vi "read_waveform.vi"(8 "error in (no error)":errorcluster, 10 "Small?":bool, 11 "Dust Event ID":i32) -> (0 "error out":errorcluster, 3 "Waveform":T1)   [LabVIEW 2013]
uses:
  Controls/Waveforms.ctl
  <vilib>/addons/h5labview/H5F_mode.ctl
  Public API/Post_Signal.ctl
  Controls/Role ID.ctl
  Controls/Hardware ID.ctl
  <userlib>/_OpenG.lib/file/file.llb/File Exists - Scalar__ogtk.vi
  <vilib>/addons/h5labview/polymorph/H5A_read_var.vi
  <vilib>/addons/database/_DB Variant To Data/Database Variant To Data.xnode
  <vilib>/addons/h5labview/H5File.lvlib
  <vilib>/addons/h5labview/H5GroupObject.lvlib
  <vilib>/addons/h5labview/H5Attrib.lvlib
panel:
  out "Query Syntax":string
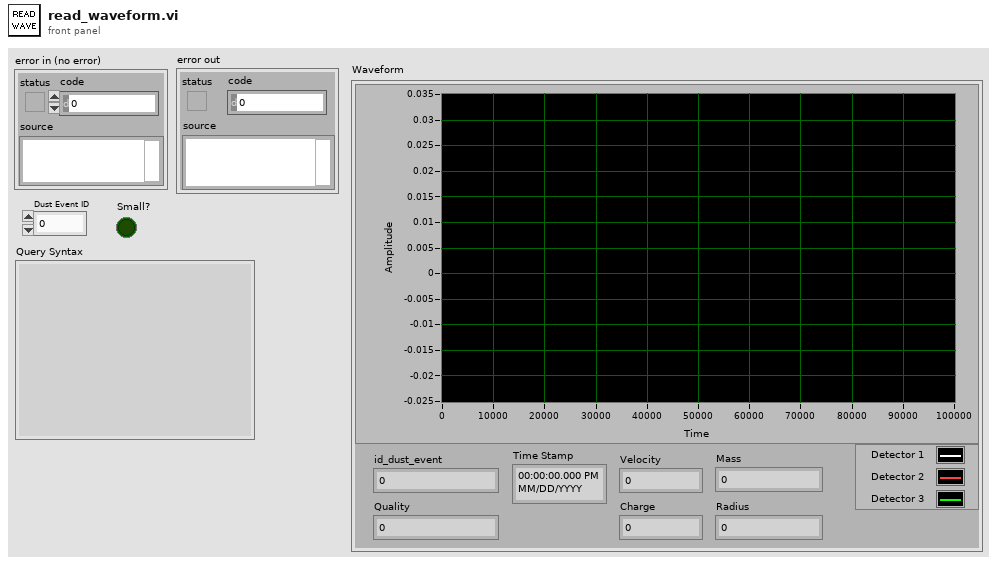
[diagram p1: front panel]
types:
  T1 = typedef "Waveforms.ctl" = cluster{"id_dust_event":u64, "Time Stamp":timestamp, "Velocity":dbl, "Mass":dbl, "Charge":dbl, "Radius":dbl, "Waveform Graph":sgl[][], "Quality":i32}
  T2 = typedef "H5File.lvlib/H5F_mode.ctl" = enum16{"read-only", "read-write", "overwrite", "create new", "open or create"}
  T3 = typedef "Role ID.ctl" = enum16{"First_Detector", "Second_Detector", "Third_Detector", "LeCroy_CH1", "LeCroy_CH2", "LeCroy_CH3", "LeCroy_CH4", "PSU"}
  T4 = typedef "Post_Signal.ctl" = cluster{"Integer Timestamp":i64, "Dust Event ID":i64, "Role ID":T3, "Data":sgl[], "Signal Length":i32, "dt":sgl, "Offset":dbl, "Hardware ID":T5}
  T5 = typedef "Hardware ID.ctl" = enum16{"Unknown", "CSA 1", "CSA 2", "CSA 3", "CSA 4", "CSA 5", "CSA 6"}
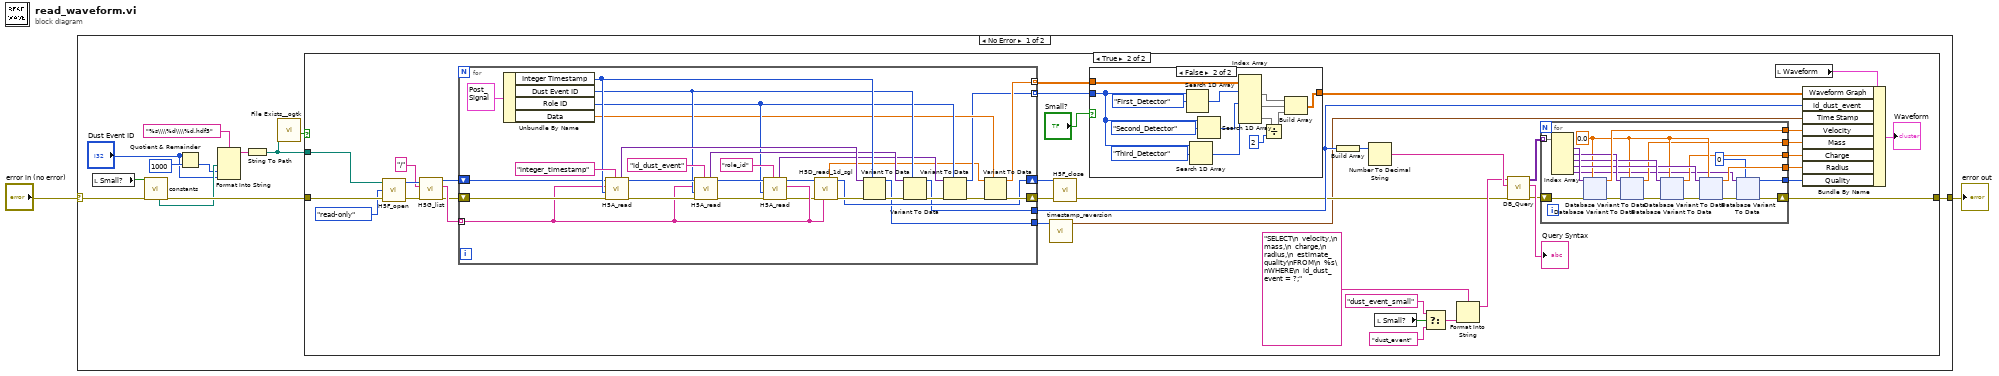
[diagram p0: block diagram]
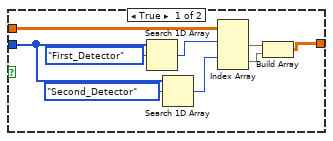
[diagram p3: hidden frame]
diagram:
  n1 = case shown="No Error" "error in (no error)" {
    selector: "error in (no error)" -> [w13 w287]
    tunnel: [w5 w287] -> w2
    frame No Error {
      n2 = local read "Small?"() -> (w6:bool)
      n3 = call "constants.vi"("error in (no error)"=w13, "Small?"=w6) -> ("error out"=w14:errorcluster, "file path for Processed Signal .hdf5 files"=w10:path)  [unwired: 4 in, 4 out]
      n4 = Quotient & Remainder(x="Dust Event ID", y=1000) -> (floor(x/y)=w9:i32)  [unwired: 1 out]
      n5 = Format Into String(format string="%s\\\\%d\\\\%d.hdf5", w10, w9, "Dust Event ID") -> (resulting string=w7:string)  [unwired: 2 in, 1 out]
      n6 = String To Path(string=w7) -> (path=w3:path)
      n7 = call-poly <userlib>:"File Exists__ogtk.vi"("file path"=w3) -> ("exists"=w4:bool)  [unwired: 6 in, 1 out]
      n8 = case shown="True" w4 {
        tunnel: w14 -> [w15 w53]
        tunnel: w3 -> [_ w52]
        tunnel: [w15 w49] -> w5
        frame False {
        }
        frame True {
          n9 = call <vilib>:"H5F_open.vi"("error in (no error)"=w53, "mode"=H5F_mode."read-only", "path"=w52) -> ("error out"=w50:errorcluster, "ref"=w48:i32)  [unwired: 1 in]
          n10 = call <vilib>:"H5G_list.vi"("error in (no error)"=w50, "group"="/", "ref"=w48) -> ("error out"=w17:errorcluster, "names"=w22:string[], "ref out"=w18:i32)  [unwired: 1 in, 1 out]
          n11 = for {
            shift-right: [w260] -> w19
            shift-left: w17 -> [w281]
            shift-right: [w259] -> w20
            shift-left: w18 -> [w282]
            tunnel: w22 -> [w265] mode=indexing
            tunnel: [w262] -> w24 mode=indexing
            tunnel: [w263] -> w25 mode=indexing
            tunnel: [w257] -> w45
            tunnel: [w258] -> w27
            n12 = Unbundle By Name(T4 {"Integer Timestamp"=0, "Dust Event ID"=0, "Role ID"=enum."First_Detector", "Data"=[], "Signal Length"=0, "dt"=0.0, "Offset"=0.0, "Hardware ID"=enum."CSA 1"} ("Post_Signal 2")) -> ("Integer Timestamp"=w284:i64, "Dust Event ID"=w276:i64, "Role ID"=w270:T3, "Data"=w267:sgl[])
            n13 = call-poly <vilib>:"H5A_read.vi"("attrib_name"="integer_timestamp", "error in (no error)"=w281, "default"=w284, "obj_name"=w265, "ref"=w282) -> ("error out"=w278:errorcluster, "ref out"=w280:i32, "value"=w283:variant)  [unwired: 2 in]
            n14 = call-poly <vilib>:"H5A_read.vi"("attrib_name"="id_dust_event", "error in (no error)"=w278, "default"=w276, "obj_name"=w265, "ref"=w280) -> ("error out"=w274:errorcluster, "ref out"=w273:i32, "value"=w277:variant)  [unwired: 2 in]
            n15 = call-poly <vilib>:"H5A_read.vi"("attrib_name"="role_id", "error in (no error)"=w274, "default"=w270, "obj_name"=w265, "ref"=w273) -> ("error out"=w264:errorcluster, "ref out"=w266:i32, "value"=w271:variant)  [unwired: 2 in]
            n16 = call "H5D_read_1d_sgl.vi"("name"=w265, "error in (no error)"=w264, "ref"=w266) -> ("error out"=w261:errorcluster, "ref out"=w259:i32, "data"=w256:sgl[])  [unwired: 4 in]
            n17 = Variant To Data(error in=w261, type=w284, Variant=w283) -> (data=w258:i64, error out=w275:errorcluster)
            n18 = Variant To Data(error in=w275, type=w276, Variant=w277) -> (data=w257:i64, error out=w269:errorcluster)
            n19 = Variant To Data(error in=w269, type=w270, Variant=w271) -> (data=w262:T3, error out=w268:errorcluster)
            n20 = Variant To Data(error in=w268, type=w267, Variant=w256) -> (data=w263:sgl[], error out=w260:errorcluster)
          }
          n21 = call "timestamp_reversion.vi"("Integer Timestamp"=w27) -> ("time stamp"=w28:timestamp)  [unwired: 8 in, 1 out]
          n22 = call <vilib>:"H5F_close.vi"("error in (no error)"=w19, "ref"=w20) -> ("error out"=w42:errorcluster)  [unwired: 3 in]
          n23 = case shown="False" "Small?" {
            tunnel: w24 -> [w238 w251]
            tunnel: w25 -> [w236 w248]
            tunnel: [w233 w245] -> w26
            frame True {
              n24 = Search 1D Array(1D array=w238, element=Role_ID."First_Detector") -> (index of element=w239:i32)  [unwired: 1 in]
              n25 = Search 1D Array(1D array=w238, element=Role_ID."Second_Detector") -> (index of element=w237:i32)  [unwired: 1 in]
              n26 = Index Array(array=w236, index (row) #1=w239, index (row) #2=w237) -> (element #1=w235:sgl[], element #2=w234:sgl[])  [unwired: 2 in]
              n27 = Build Array(w235, w234) -> (w233:sgl[][])
            }
            frame False {
              n28 = Search 1D Array(1D array=w251, element=Role_ID."First_Detector") -> (index of element=w253:i32)  [unwired: 1 in]
              n29 = Search 1D Array(1D array=w251, element=Role_ID."Third_Detector") -> (index of element=w249:i32)  [unwired: 1 in]
              n30 = Search 1D Array(1D array=w251, element=Role_ID."Second_Detector") -> (index of element=w250:i32)  [unwired: 1 in]
              n31 = Index Array(array=w248, index (row) #1=w253, index (row) #2=w250, index (row) #3=w249) -> (element #1=w247:sgl[], element #2=w246:sgl[], element #3=w244:sgl[])  [unwired: 3 in]
              n32 = Divide(x=w244, y=2 ("Numeric")) -> (x/y=w243:sgl[])
              n33 = Build Array(w247, w246, w243) -> (w245:sgl[][])
            }
          }
          n34 = Build Array(w45) -> (w46:i64[])
          n35 = Number To Decimal String(number=w46) -> (decimal integer string=w47:string[])  [unwired: 1 in]
          n36 = local read "Small?"() -> (w32:bool)
          n37 = Select(t="dust_event_small" ("resulting string"), s=w32, f="dust_event" ("resulting string")) -> (s? t:f=w31:string)
          n38 = Format Into String(format string="SELECT\n  velocity,\n  mass,\n  charge,\n  radius,\n  estimate_quality\nFROM\n  %s\nWHERE\n  id_dust_event = ?;" ("SQL query"), w31) -> (resulting string=w44:string)  [unwired: 2 in, 1 out]
          n39 = call "DB_Query.vi"("error in (no error)"=w42, "Parameters"=w47, "Parameterized Query"=w44) -> ("error out"=w40:errorcluster, "Query in Standard Format"=→"Query Syntax":string, "Results"=w41:variant[][])  [unwired: 6 in]
          n40 = for {
            tunnel: w41 -> [w71] mode=indexing
            shift-right: [w57] -> w49
            shift-left: w40 -> [w72]
            tunnel: [w68] -> w35
            tunnel: [w61] -> w36
            tunnel: [w60] -> w37
            tunnel: [w59] -> w38
            tunnel: [w54] -> w39
            w62 = 0.0 ("Velocity")
            n41 = Index Array(array=w71) -> (element #1=w70:variant, element #2=w67:variant, element #3=w65:variant, element #4=w63:variant, element #5=w56:variant)  [unwired: 5 in]
            n42 = xnode "Database Variant To Data"("database variant"=w70, "error in (no error)"=w72, "type"=w62) -> ("data"=w68:dbl, "error out"=w69:errorcluster)
            n43 = xnode "Database Variant To Data"("database variant"=w67, "error in (no error)"=w69, "type"=w62) -> ("data"=w61:dbl, "error out"=w66:errorcluster)
            n44 = xnode "Database Variant To Data"("database variant"=w65, "error in (no error)"=w66, "type"=w62) -> ("data"=w60:dbl, "error out"=w64:errorcluster)
            n45 = xnode "Database Variant To Data"("database variant"=w63, "error in (no error)"=w64, "type"=w62) -> ("data"=w59:dbl, "error out"=w58:errorcluster)
            n46 = xnode "Database Variant To Data"("database variant"=w56, "error in (no error)"=w58, "type"=i64 0 ("Dust Event ID")) -> ("data"=w54:i64, "error out"=w57:errorcluster)
          }
          n47 = local read "Waveform"() -> (w23:T1)
          n48 = Bundle By Name(cluster=w23, "Waveform Graph"=w26, "id_dust_event"=w45, "Time Stamp"=w28, "Velocity"=w35, "Mass"=w36, "Charge"=w37, "Radius"=w38, "Quality"=w39) -> (→"Waveform":T1)
        }
      }
    }
    frame Error {
    }
  }
  "error out" <- w2
